vi "MSA - Prelucrare date - doar anumite componente.vi"() -> ()   [LabVIEW 2018]
uses:
  <vilib>/gmath/NI_Gmath.lvlib
panel:
  in  "Valoarea cu care se inlocuieste":dbl=2.0
  in  "Toleranta Maxima admisa %":dbl=5.0
  in  "Modificati componentele":bool
  in  "Componentele care se modifica":string[](array[string])
  out "Locatia fisierelor modificate":path
  out "Tabel cu valorile care se vor scrie in loguri":string[][](array[string])
  in  "Locatia fisierelor originale":path=path "C:/Users/q74808/Desktop/Labview facute/MAS/Ultima versiune/1x50Original"
  # "Verde: Se modifica doar anumite componente"
  # "Rosu = Se modifica toate componentele"
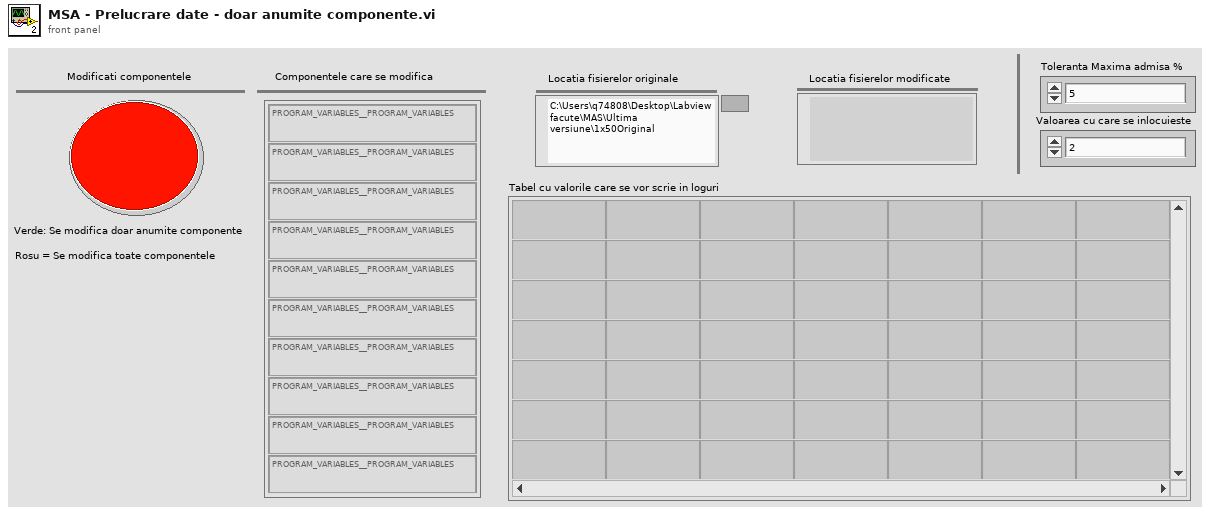
[diagram p1: front panel]
types:
  T1 = enum16{"arithmetic", "geometric", "harmonic", "trimmed", "median"}
  T2 = enum16{"open", "replace", "create", "open or create", "replace or create", "replace or create with confirmation"}
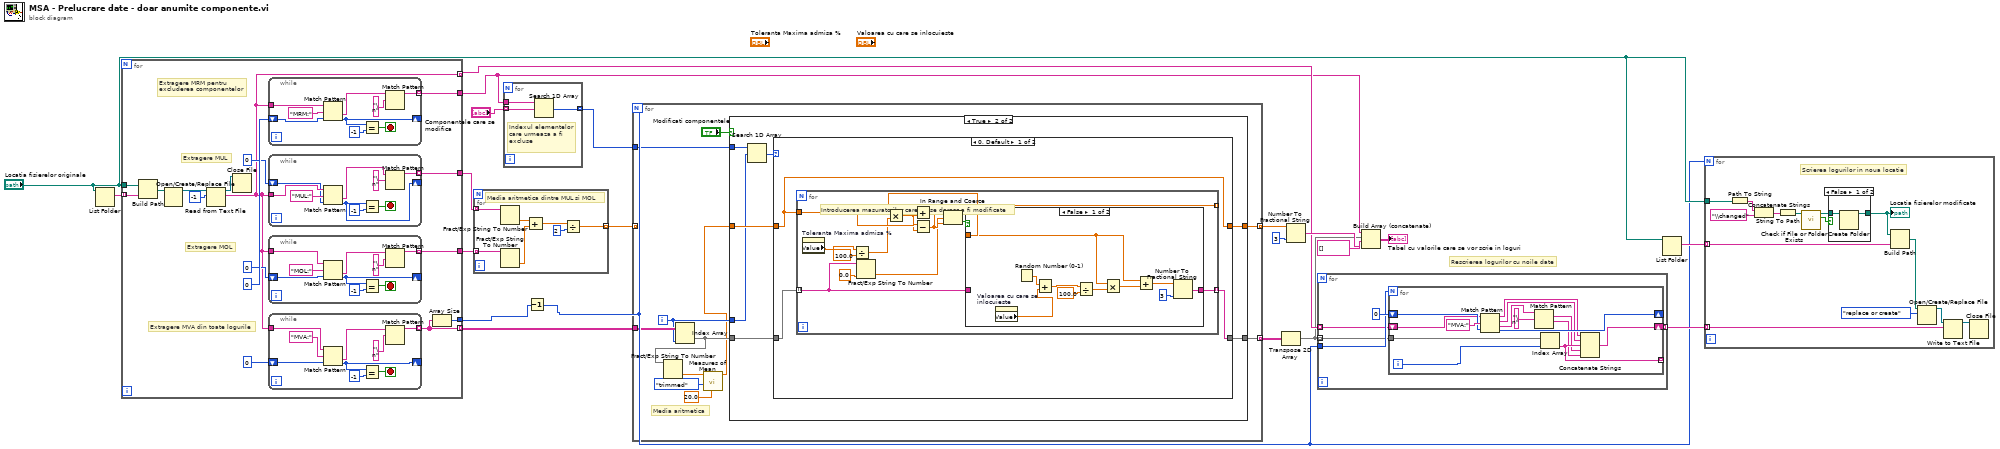
[diagram p0: block diagram]
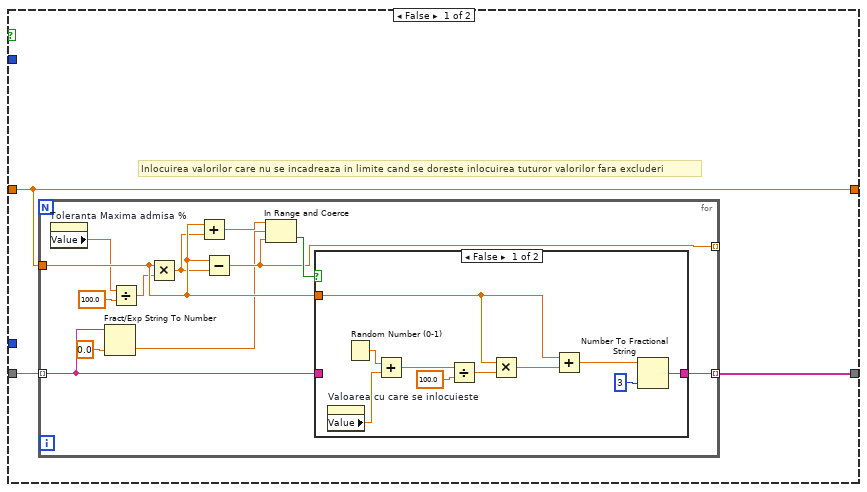
[diagram p3: hidden frame]
diagram:
  # "Rescrierea logurilor cu noile date"
  n1 = List Folder(path="Locatia fisierelor originale") -> (filenames=w21:string[])  [unwired: 3 in, 3 out]
  n2 = for {
    tunnel: w21 -> [w36] mode=indexing
    tunnel: "Locatia fisierelor originale" -> [w37]
    tunnel: [w30] -> w5
    tunnel: [w29] -> w13 mode=indexing
    tunnel: [w28] -> w2
    tunnel: [w22] -> w12 mode=indexing
    tunnel: [w25] -> w9
    tunnel: [w23] -> w10
    # "Extragere MRM pentru \nexcluderea componentelor"
    # "Extragere MUL"
    # "Extragere MOL"
    # "Extragere MVA din toate logurile"
    n3 = Build Path(base path=w37, name or relative path=w36) -> (appended path=w35:path)
    n4 = Open/Create/Replace File(file path (use dialog)=w35) -> (refnum out=w34:refnum<file>)  [unwired: 5 in, 2 out]
    n5 = Read from Text File(file (use dialog)=w34, count=-1) -> (refnum out=w27:refnum<file>, text=w22:string)  [unwired: 2 in, 2 out]
    n6 = Close File(refnum=w27) -> ()  [unwired: 1 in, 2 out]
    n7 = while {
      tunnel: w22 -> [w73]
      tunnel: [w69] -> w30 mode=indexing
      shift-right: [w66] -> _
      shift-left: 0 -> [w68]
      stop <- w67 stop-if-true
      n8 = Match Pattern(string=w73, regular expression="MRM:", offset (0)=w68) -> (after substring=w71:string, offset past match=w66:i32)  [unwired: 2 out]
      n9 = Equal?(x=w66, y=-1) -> (x = y?=w67:bool)
      n10 = Match Pattern(string=w71, regular expression="\n") -> (before substring=w69:string)  [unwired: 1 in, 3 out]
    }
    n11 = while {
      tunnel: w22 -> [w55]
      tunnel: [w51] -> w23 mode=indexing
      shift-right: [w48] -> _
      shift-left: 0 -> [w50]
      stop <- w49 stop-if-true
      n12 = Match Pattern(string=w55, regular expression="MUL:", offset (0)=w50) -> (after substring=w53:string, offset past match=w48:i32)  [unwired: 2 out]
      n13 = Equal?(x=w48, y=-1) -> (x = y?=w49:bool)
      n14 = Match Pattern(string=w53, regular expression="\n") -> (before substring=w51:string)  [unwired: 1 in, 3 out]
    }
    n15 = while {
      tunnel: w22 -> [w64]
      tunnel: [w60] -> w25 mode=indexing
      shift-right: [w57] -> _
      shift-left: 0 -> [w59]
      stop <- w58 stop-if-true
      n16 = Match Pattern(string=w64, regular expression="MOL:", offset (0)=w59) -> (after substring=w62:string, offset past match=w57:i32)  [unwired: 2 out]
      n17 = Equal?(x=w57, y=-1) -> (x = y?=w58:bool)
      n18 = Match Pattern(string=w62, regular expression="\n") -> (before substring=w60:string)  [unwired: 1 in, 3 out]
    }
    n19 = while {
      tunnel: w22 -> [w46]
      tunnel: [w42] -> w29 mode=indexing
      shift-right: [w40] -> _
      shift-left: 0 -> [w41]
      stop <- w38 stop-if-true
      n20 = Match Pattern(string=w46, regular expression="MVA:", offset (0)=w41) -> (after substring=w44:string, offset past match=w40:i32)  [unwired: 2 out]
      n21 = Equal?(x=w40, y=-1) -> (x = y?=w38:bool)
      n22 = Match Pattern(string=w44, regular expression="\n") -> (before substring=w42:string)  [unwired: 1 in, 3 out]
    }
    n23 = Array Size(array=w29) -> (size(s)=w28:i32)
  }
  n24 = for {
    tunnel: w10 -> [w80] mode=indexing
    tunnel: w9 -> [w79] mode=indexing
    tunnel: [w75] -> w8 mode=indexing
    # "Media aritmetica dintre MUL si MOL"
    n25 = Fract/Exp String To Number(string=w80) -> (number=w78:dbl)  [unwired: 3 in, 1 out]
    n26 = Fract/Exp String To Number(string=w79) -> (number=w77:dbl)  [unwired: 3 in, 1 out]
    n27 = Add(x=w78, y=w77) -> (x+y=w76:dbl)
    n28 = Divide(x=w76, y=2) -> (x/y=w75:dbl)
  }
  n29 = for {
    tunnel: "Componentele care se modifica" -> [w82] mode=indexing
    tunnel: w5 -> [w83]
    tunnel: [w81] -> w4 mode=indexing
    # "Indexul elementelor care urmeaza a fi excluse"
    n30 = Search 1D Array(1D array=w83, element=w82) -> (index of element=w81:i32)  [unwired: 1 in]
  }
  n31 = Decrement(x=w2) -> (x-1=w1:i32)
  n32 = for {
    N: w1 -> [_]
    tunnel: w13 -> [w94]
    tunnel: [w89] -> w18 mode=indexing
    tunnel: [w93] -> w15 mode=indexing
    tunnel: w8 -> [_] mode=indexing
    tunnel: w4 -> [w91]
    i -> [w90]
    # "Media aritmetica"
    n33 = Index Array(array=w94, index (col)=w90) -> (element=w85:string[])  [unwired: 1 in]
    n34 = Fract/Exp String To Number(string=w85) -> (number=w88:dbl[])  [unwired: 3 in, 1 out]
    n35 = call <vilib>:"Measures of Mean.vi"("percent (trim)"=20.0, "type"=T1."trimmed", "x array"=w88) -> ("mean value"=w84:dbl)  [unwired: 7 in, 1 out]
    n36 = case shown="True" "Modificati componentele" {
      tunnel: [w96 w127] -> w93
      tunnel: w84 -> [w95 w125]
      tunnel: w85 -> [w97 w126]
      tunnel: w91 -> [_ w123]
      tunnel: w90 -> [_ w122]
      tunnel: [w95 w124] -> w89
      frame False {
        # "Inlocuirea valorilor care nu se incadreaza in limite cand se doreste inlocuirea tuturor valorilor fara excluderi"
        n37 = for {
          tunnel: w95 -> [w106]
          tunnel: w97 -> [w108] mode=indexing
          tunnel: [w107] -> w96 mode=indexing
          tunnel: [w103] -> _ mode=indexing
          n38 = property on="Toleranta Maxima admisa %" class="DigNum (strict)"() -> ("Value"=w98:dbl)  [unwired: 2 in, 2 out]
          n39 = Fract/Exp String To Number(string=w108, default (0 dbl)=0.0) -> (number=w101:dbl)  [unwired: 2 in, 1 out]
          n40 = Divide(x=w98, y=100.0) -> (x/y=w99:dbl)
          n41 = Multiply(x=w106, y=w99) -> (x*y=w105:dbl)
          n42 = Add(x=w106, y=w105) -> (x+y=w104:dbl)
          n43 = Subtract(x=w106, y=w105) -> (x-y=w103:dbl)
          n44 = In Range and Coerce(upper limit=w104, x=w101, lower limit=w103) -> (In Range?=w109:bool)  [unwired: 1 out]
          n45 = case shown="False" w109 {
            tunnel: w108 -> [_ w120]
            tunnel: [w116 w120] -> w107
            tunnel: w106 -> [w119 _]
            frame False {
              n46 = property on="Valoarea cu care se inlocuieste" class="DigNum (strict)"() -> ("Value"=w110:dbl)  [unwired: 2 in, 2 out]
              n47 = Random Number (0-1)() -> (number: 0 to 1=w112:dbl)
              n48 = Add(x=w112, y=w110) -> (x+y=w111:dbl)
              n49 = Divide(x=w111, y=100.0) -> (x/y=w114:dbl)
              n50 = Multiply(x=w119, y=w114) -> (x*y=w118:dbl)
              n51 = Add(x=w119, y=w118) -> (x+y=w117:dbl)
              n52 = Number To Fractional String(number=w117, precision (6)=i16 3) -> (F-format string=w116:string)  [unwired: 2 in]
            }
            frame True {
            }
          }
        }
      }
      frame True {
        n53 = Search 1D Array(1D array=w123, element=w122) -> (index of element=w121:i32)  [unwired: 1 in]
        n54 = case shown="0, Default" w121 {
          tunnel: [w128 w154] -> w127
          tunnel: w125 -> [w130 w155]
          tunnel: w126 -> [w129 w154]
          tunnel: [w130 w155] -> w124
          frame 0, Default {
            # "Introducerea masuratorilor care nu se doresc a fi modificate"
            n55 = for {
              tunnel: w130 -> [w139]
              tunnel: w129 -> [w141] mode=indexing
              tunnel: [w140] -> w128 mode=indexing
              tunnel: [w136] -> _ mode=indexing
              n56 = property on="Toleranta Maxima admisa %" class="DigNum (strict)"() -> ("Value"=w131:dbl)  [unwired: 2 in, 2 out]
              n57 = Divide(x=w131, y=100.0) -> (x/y=w132:dbl)
              n58 = Fract/Exp String To Number(string=w141, default (0 dbl)=0.0) -> (number=w134:dbl)  [unwired: 2 in, 1 out]
              n59 = Multiply(x=w139, y=w132) -> (x*y=w138:dbl)
              n60 = Add(x=w139, y=w138) -> (x+y=w137:dbl)
              n61 = Subtract(x=w139, y=w138) -> (x-y=w136:dbl)
              n62 = In Range and Coerce(upper limit=w137, x=w134, lower limit=w136) -> (In Range?=w142:bool)  [unwired: 1 out]
              n63 = case shown="False" w142 {
                tunnel: w141 -> [_ w153]
                tunnel: [w149 w153] -> w140
                tunnel: w139 -> [w152 _]
                frame False {
                  n64 = property on="Valoarea cu care se inlocuieste" class="DigNum (strict)"() -> ("Value"=w143:dbl)  [unwired: 2 in, 2 out]
                  n65 = Random Number (0-1)() -> (number: 0 to 1=w145:dbl)
                  n66 = Add(x=w145, y=w143) -> (x+y=w144:dbl)
                  n67 = Divide(x=w144, y=100.0) -> (x/y=w147:dbl)
                  n68 = Multiply(x=w152, y=w147) -> (x*y=w151:dbl)
                  n69 = Add(x=w152, y=w151) -> (x+y=w150:dbl)
                  n70 = Number To Fractional String(number=w150, precision (6)=i16 3) -> (F-format string=w149:string)  [unwired: 2 in]
                }
                frame True {
                }
              }
            }
          }
          frame -1 {
            # "Introducerea masuratorilor care se doresc a fi modificate"
          }
        }
      }
    }
  }
  n71 = Transpose 2D Array(2D array=w15) -> (transposed array=w11:string[][])
  n72 = Number To Fractional String(number=w18, precision (6)=i16 3) -> (F-format string=w17:string[])  [unwired: 2 in]
  n73 = for {
    tunnel: w1 -> [w159]
    tunnel: w12 -> [w158] mode=indexing
    tunnel: w11 -> [w157] mode=indexing
    tunnel: [w156] -> w3 mode=indexing
    n74 = for {
      N: w159 -> [_]
      shift-right: [w171] -> _
      shift-left: 0 -> [w172]
      tunnel: w157 -> [w169]
      tunnel: [w165] -> _ mode=indexing
      shift-right: [w163] -> w156
      shift-left: w158 -> [w168]
      i -> [w161]
      n75 = Match Pattern(string=w168, regular expression="MVA:", offset (0)=w172) -> (before substring=w167:string, match substring=w166:string, after substring=w170:string, offset past match=w171:i32)
      n76 = Match Pattern(string=w170, regular expression="\n") -> (match substring=w164:string, after substring=w162:string)  [unwired: 1 in, 2 out]
      n77 = Index Array(array=w169, index=w161) -> (element=w165:string)
      n78 = Concatenate Strings(w167, w166, w165, w164, w162) -> (w163:string)
    }
  }
  n79 = Build Array (concatenate)(w5, w11, string[] [] ("element"), w17) -> (→"Tabel cu valorile care se vor scrie in loguri":string[][])
  n80 = List Folder(path="Locatia fisierelor originale") -> (filenames=w14:string[])  [unwired: 3 in, 3 out]
  n81 = for {
    N: w1 -> [_]
    tunnel: "Locatia fisierelor originale" -> [w185]
    tunnel: w14 -> [w188] mode=indexing
    tunnel: w3 -> [w181] mode=indexing
    # "Scrierea logurilor in noua locatie"
    n82 = Path To String(path=w185) -> (string=w184:string)
    n83 = Concatenate Strings(w184, "\\changed") -> (w179:string)
    n84 = String To Path(string=w179) -> (path=w178:path)
    n85 = call <vilib>:"Check if File or Folder Exists.vi"("path"=w178) -> ("file or folder exists?"=w177:bool, "dup path"=w176:path)  [unwired: 8 in, 1 out]
    n86 = case shown="False" w177 {
      tunnel: w176 -> [w190 w191]
      tunnel: [w189 w191] -> w175
      frame False {
        n87 = Create Folder(path (use dialog)=w190) -> (created path=w189:path)  [unwired: 2 in, 2 out]
      }
      frame True {
      }
    }
    "Locatia fisierelor modificate" <- w175
    n88 = Build Path(base path=w175, name or relative path=w188) -> (appended path=w186:path)
    n89 = Open/Create/Replace File(file path (use dialog)=w186, operation (0:open)=T2."replace or create") -> (refnum out=w182:refnum<file>)  [unwired: 4 in, 2 out]
    n90 = Write to Text File(file (use dialog)=w182, text=w181) -> (refnum out=w180:refnum<file>)  [unwired: 2 in, 2 out]
    n91 = Close File(refnum=w180) -> ()  [unwired: 1 in, 2 out]
  }
